vi "0_StageToStave.vi"(0 "Image feed":T1(plugin-control), 1 "Stave origin in XYZ Frame":T2, 2 "Stave Coordinate System":enum16{"Tooling Pins", "Bus Tape"}(ring), 3 "Pixel resolution [um/pix]":dbl=3.5 format="%#_13g", 4 "Axes Speeds [mm/s]":T3={"X Speed"=25.0, "Y Speed"=10.0, "Z Speed"=10.0}, 5 "N pics captured":i32=10, 6 "Pause before image capture [ms]":u32=3500, 7 "error in":errorcluster, 9 "Record keeping file path":path=path "E:/XYZstage+Camera_CollectedImages/12-22-2016/images", 11 "XYZ .NET Refnum in":refnum<k24>, 12 "Autofocus Coord in XYZ Frame":T2, 13 "Current Build Phase":refnum<vi>, 14 "Templates path":path=path "C:/Users/Sciolla Lab/Desktop/BNLStaveAssembly-Laura/edgeimagebig.png", 26 "Calibration Results":refnum<vi>) -> (15 "Cross- check: Are these the center of pins in the center of the image?":T1[](array[plugin-control])=["remote image 000000001396EDEC", "remote image 000000001392CD9C", "remote image 000000001392D204", "remote image 00000000139777D4", "remote image 000000001397783C", "image_5", "image_6", "image_7", "image_8", "image_9", "image_10", "image_11", "image_12", "image_13", "image_14", "image_15", "image_16", "image_17"], 16 "Finished!":bool, 17 "Check: Plot of average point in each pin":T4(graph), 19 "XYZ .NET Refnum out":refnum<k24>, 21 "Angle of pins [rad]":dbl, 24 "Calibrated stave origin (X,Y) [mm]":dbl[](array[numeric]), 25 "Calibrated stave basis [mm]":dbl[][](array[numeric]), 27 "Error report":errorcluster)   [LabVIEW 2016]
uses:
  C:/Users/Aerotech/Documents/BNL_ThermomechanicalStave/AerotechLibraries/Bin/Aerotech.A3200.dll
  AerotechLibraries/Bin/Aerotech.A3200.dll
  <vilib>/Utility/file.llb/Write Delimited Spreadsheet (DBL).vi
panel:
  out "Image Array":T1[](array[plugin-control])=["remote image 000000001396EDEC", "remote image 000000001392CD9C", "remote image 000000001392D204", "remote image 00000000139777D4", "remote image 000000001397783C", "image_5", "image_6", "image_7", "image_8", "image_9", "image_10", "image_11", "image_12", "image_13", "image_14", "image_15", "image_16", "image_17"]
  out "Stave Z [mm]":dbl
  out "Ideal pin locations":dbl[][](array[numeric])
  # "RESULTS"
  # "CONTROLS"
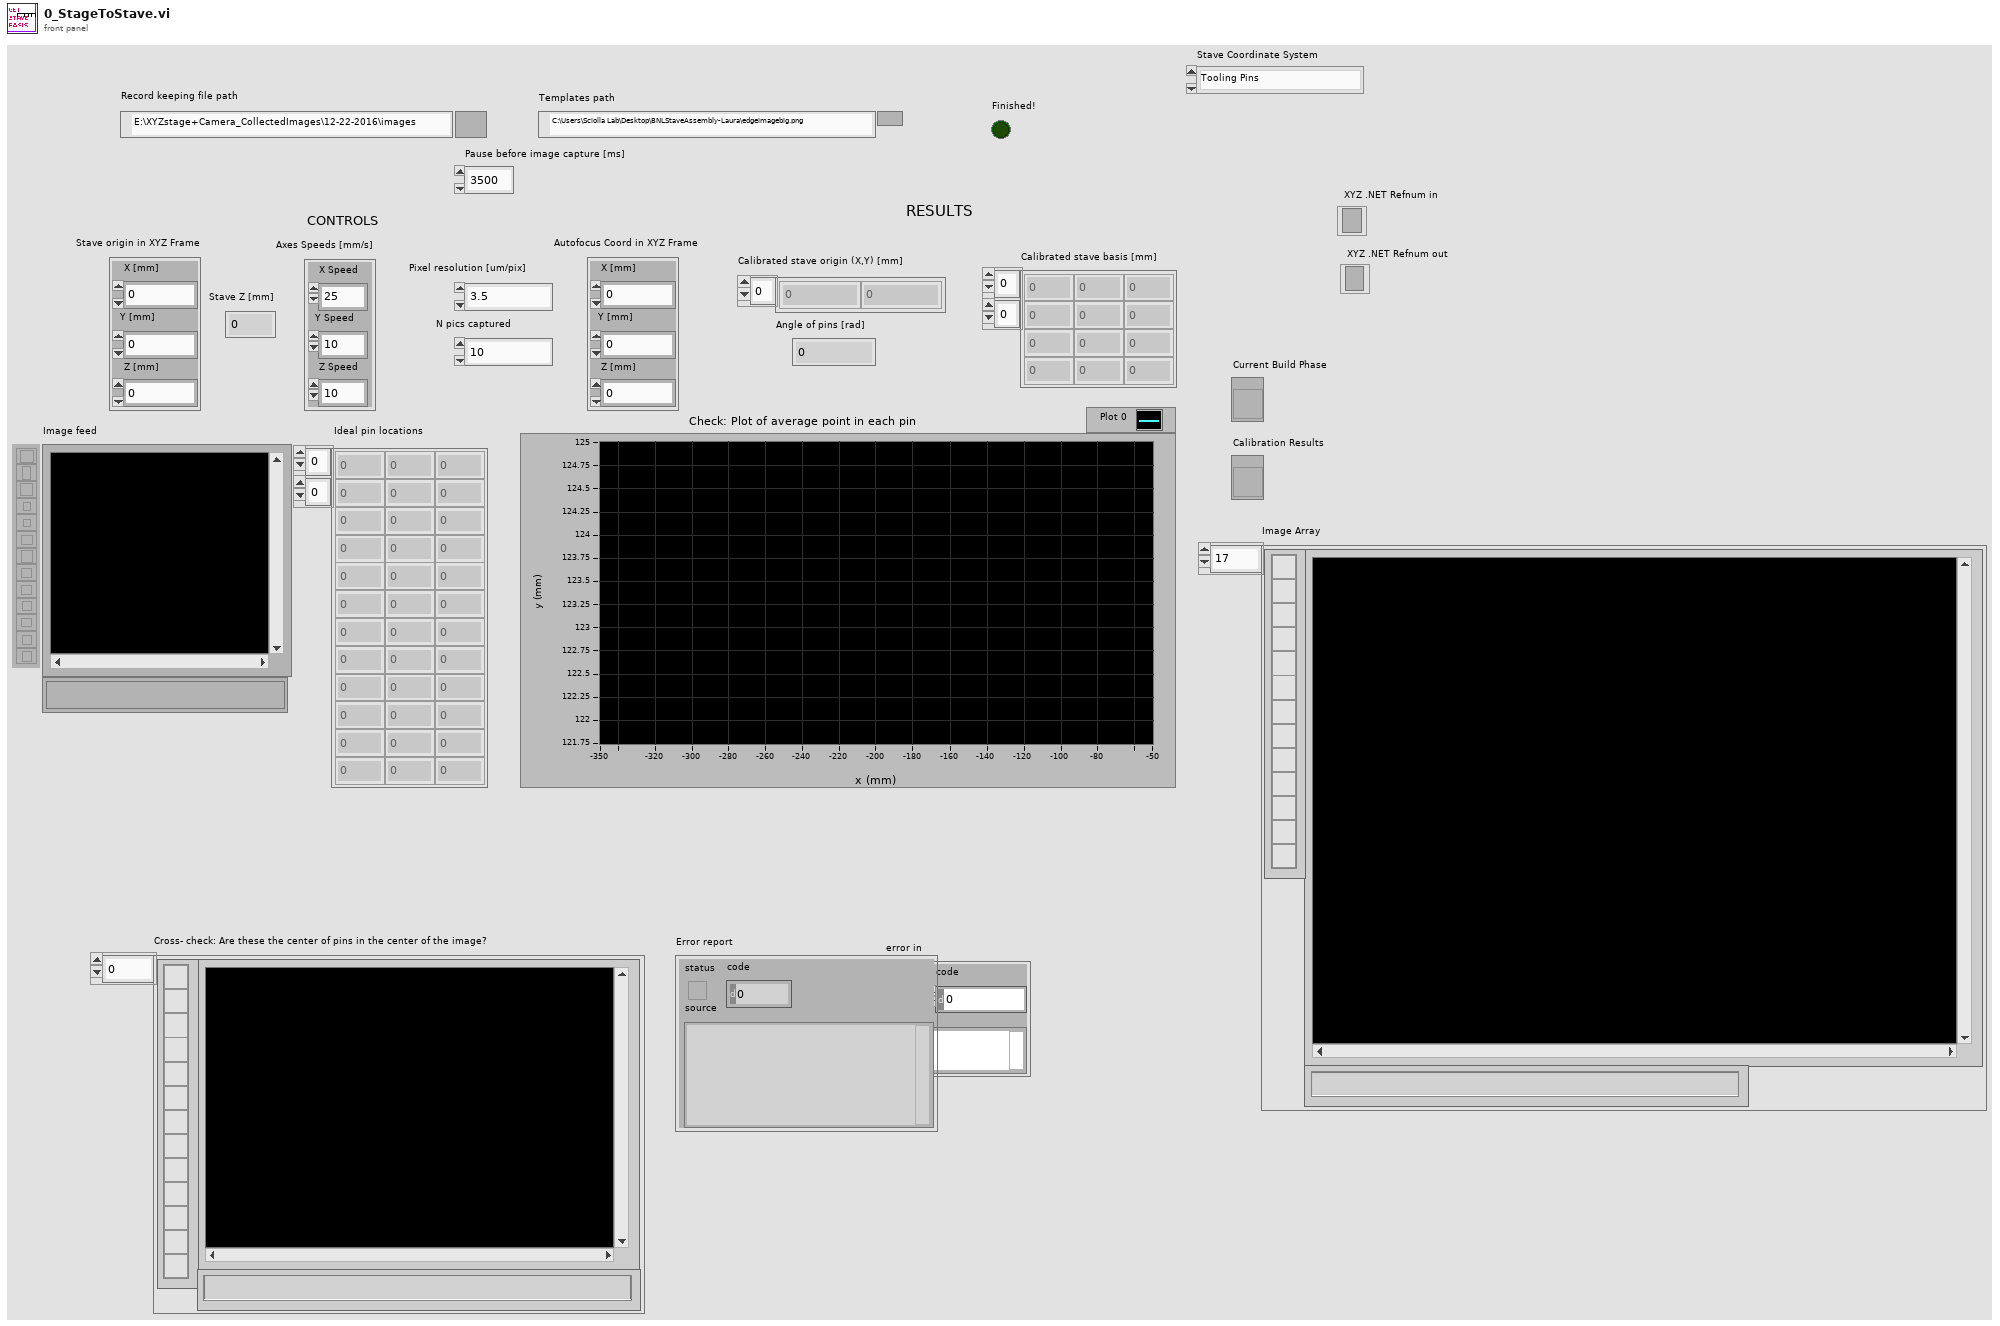
[diagram p1: front panel]
types:
  T1 = typedef "IMAQ Image.ctl" = refnum<image>
  T2 = cluster{"X [mm]":dbl, "Y [mm]":dbl, "Z [mm]":dbl}
  T3 = cluster{"X Speed":dbl, "Y Speed":dbl, "Z Speed":dbl}
  T4 = cluster{"Top averages":dbl[], "Best Linear Fit":dbl[]}[]
  T5 = cluster{"Image feed":T1, "Axes Speeds [mm/s]":cluster{"X Speed":dbl, "Y Speed":dbl, "Z Speed":dbl}, "XYZ .NET Refnum in":refnum<k24>}
  T6 = cluster{"Captured positions":dbl[][], "XYZ .NET Refnum out":refnum<k24>}
  T7 = cluster{"Camera calibration results":cluster{"Calibration [um/pix]":dbl, "Working distance to stave [mm]":dbl, "Calib uncertainty [um/pix]":dbl, "WD Uncertainty [mm]":dbl}, "Stave basis calibration results":cluster{"Angle, stave & xyz stage [rad]":dbl, "Calibrated stave origin (X,Y) [mm]":dbl[]}}
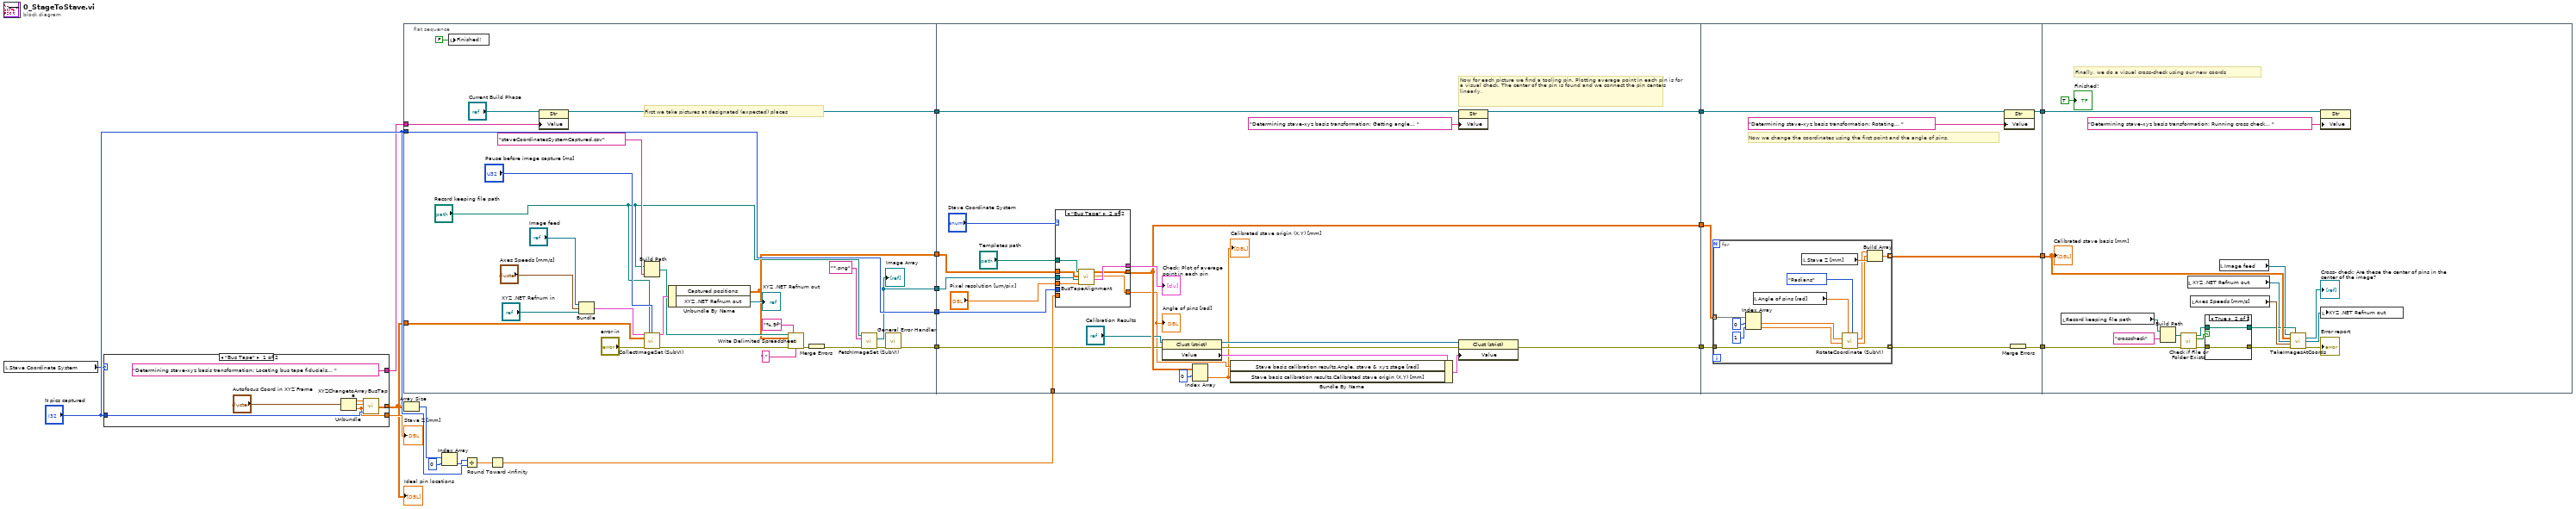
[diagram p0: block diagram]
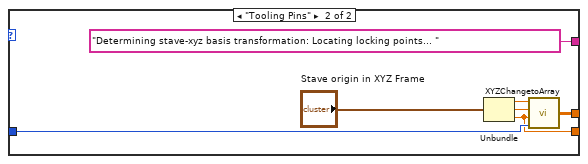
[diagram p2: hidden frame]
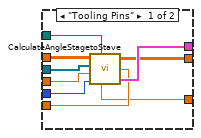
[diagram p3: hidden frame]
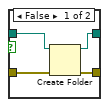
[diagram p4: hidden frame]
diagram:
  n1 = local read "Stave Coordinate System"() -> (w2:enum16{"Tooling Pins", "Bus Tape"})
  n2 = case shown="\"Bus Tape\"" w2 {
    tunnel: "N pics captured" -> [w25 w33]
    tunnel: [w23 w30] -> w8
    tunnel: [w24 w32] -> w3
    tunnel: ["Determining stave-xyz basis transformation: Locating bus tape fiducials... " ("Value") "Determining stave-xyz basis transformation: Locating locking points... " ("Value")] -> w1
    frame "Bus Tape" {
      n3 = Unbundle("Autofocus Coord in XYZ Frame") -> ("X [mm]"=w27:dbl, "Y [mm]"=w26:dbl, "Z [mm]"=w23:dbl)
      n4 = call "XYZChangetoArrayBusTape.vi"("N pics captured"=w25, "z change"=w23, "y change"=w26, "x change"=w27) -> ("Array of Coords to go to"=w24:dbl[][])  [unwired: 2 in]
    }
    frame "Tooling Pins" {
      n5 = Unbundle("Stave origin in XYZ Frame") -> ("X [mm]"=w35:dbl, "Y [mm]"=w34:dbl, "Z [mm]"=w30:dbl)
      n6 = call "XYZChangetoArray.vi"("N pics captured"=w33, "z change"=w30, "y change"=w34, "x change"=w35) -> ("Array of Coords to go to"=w32:dbl[][])  [unwired: 2 in]
    }
  }
  "Ideal pin locations" <- w3
  "Stave Z [mm]" <- w8
  n7 = flat-sequence {
    tunnel: [w43] -> w19
    tunnel: [w42] -> w17
    tunnel: [w44] -> w16
    tunnel: w3 -> [w47]
    tunnel: "N pics captured" -> [w62]
    tunnel: [w62] -> w15
    tunnel: [w59] -> w7
    tunnel: w1 -> [w37]
    tunnel: [w82] -> w21
    tunnel: w19 -> [w81]
    tunnel: [w68] -> w18
    tunnel: w17 -> [w69]
    tunnel: w16 -> [w79]
    tunnel: w15 -> [w77]
    tunnel: w9 -> [w76]
    tunnel: w7 -> [w74]
    tunnel: [w73] -> w6
    tunnel: w21 -> [w108]
    tunnel: [w107] -> w20
    tunnel: w18 -> [w103]
    tunnel: w6 -> [w105]
    tunnel: [w104] -> w5
    tunnel: [w101] -> w4
    tunnel: w20 -> [w140]
    tunnel: w5 -> [w127]
    tunnel: w4 -> [w126]
    frame #0 {
      # "First we take pictures at designated (expected) places"
      n8 = local write "Finished!"(FALSE) -> ()
      n9 = property class="Str"(reference="Current Build Phase", "Value"=w37) -> (reference out=w59:refnum<vi>)  [unwired: 1 in, 1 out]
      n10 = Bundle("Image feed"="Image feed", "Axes Speeds [mm/s]"="Axes Speeds [mm/s]", "XYZ .NET Refnum in"="XYZ .NET Refnum in") -> (w40:T5)  [unwired: 1 in]
      n11 = Build Path(base path="Record keeping file path", name or relative path="staveCoordinatesSystemCaptured.csv") -> (appended path=w50:path)
      n12 = call "CollectImageSet (SubVI).vi"("Inputs"=w40, "Path to save collected images"="Record keeping file path", "milliseconds to wait"="Pause before image capture [ms]", "Set of coordinates to process"=w47, "error in"="error in") -> ("Outputs"=w54:T6, "error out"=w56:errorcluster)  [unwired: 8 in, 1 out]
      n13 = Unbundle By Name(w54) -> ("Captured positions"=w44:dbl[][], "XYZ .NET Refnum out"=→"XYZ .NET Refnum out":refnum<k24>)
      n14 = call-poly <vilib>:"Write Delimited Spreadsheet.vi"("file path (dialog if empty)"=w50, "format (%.3f)"="%.9f", "2D data"=w44, "error in (no error)"=w56, "delimiter (\\t)"="," ("delimiter (\\t)")) -> ("error out"=w55:errorcluster)  [unwired: 9 in, 1 out]
      n15 = Merge Errors(w55) -> (w52:errorcluster)
      n16 = call "FetchImageSet (SubVI).vi"("error in (no error)"=w52, "Naming Convention"="*.png", "Images Directory"="Record keeping file path") -> ("error out"=w51:errorcluster, "Image Array"=w43:T1[])  [unwired: 6 in, 1 out]
      "Image Array" <- w43
      n17 = call <vilib>:"General Error Handler.vi"("error in (no error)"=w51) -> ("error out"=w42:errorcluster)  [unwired: 2 in, 12 out]
    }
    frame #1 {
      # "Now for each picture we find a tooling pin. Plotting average point in each pin is for a visual check. The center of the pin is found and we connect the pin centers linearly."
      n18 = case shown="\"Bus Tape\"" "Stave Coordinate System" {
        tunnel: [w93 w96] -> w84
        tunnel: [w92 w95] -> w82
        tunnel: w81 -> [w91 w98]
        tunnel: "Pixel resolution [um/pix]" -> [w90 w97]
        tunnel: w79 -> [w89 w99]
        tunnel: "Templates path" -> [w88 w100]
        tunnel: w77 -> [w87 _]
        tunnel: w76 -> [w86 _]
        tunnel: [w85 w94] -> w66
        frame "Tooling Pins" {
          n19 = call "CalculateAngleStagetoStave.vi"("Coordinates from images"=w89, "Templates path"=w88, "Image Array"=w91, "Pixel resolution"=w90, "Number of images each"=w87, "Number of pins"=w86) -> ("Angle"=w85:dbl, "Locations pins"=w92:dbl[][], "Each point on located edges"=w93:T4)
        }
        frame "Bus Tape" {
          n20 = call "BusTapeAlignment.vi"("um/pix resolution"=w97, "Input Images Array"=w98, "Input Coordinate Array"=w99, "Template Path"=w100) -> ("Bus Tape Positions"=w96:cluster{"Top":dbl[], "Top":dbl[]}[], "Angle (rad)"=w94:dbl, "Average positions"=w95:dbl[][])  [unwired: 4 in, 1 out]
        }
      }
      "Check: Plot of average point in each pin" <- w84
      "Angle of pins [rad]" <- w66
      n21 = property class="Clust (strict)"(reference="Calibration Results", error in=w69) -> (reference out=w71:refnum<vi>, error out=w70:errorcluster, "Value"=w67:T7)
      n22 = Index Array(array=w82, index (row)=0) -> (element=w65:dbl[])  [unwired: 1 in]
      "Calibrated stave origin (X,Y) [mm]" <- w65
      n23 = Bundle By Name(cluster=w67, "Stave basis calibration results.Angle, stave & xyz stage [rad]"=w66, "Stave basis calibration results.Calibrated stave origin (X,Y) [mm]"=w65) -> (w64:T7)
      n24 = property class="Str"(reference=w74, "Value"="Determining stave-xyz basis transformation: Getting angle... ") -> (reference out=w73:refnum<vi>)  [unwired: 1 in, 1 out]
      n25 = property class="Clust (strict)"(reference=w71, error in=w70, "Value"=w64) -> (error out=w68:errorcluster)  [unwired: 1 out]
    }
    frame #2 {
      # "Now we change the coordinates using the first point and the angle of pins."
      n26 = for {
        tunnel: w108 -> [w119] mode=indexing
        tunnel: [w116] -> w107 mode=indexing
        tunnel: w103 -> [w110]
        tunnel: [w109] -> w102 mode=indexing
        n27 = Index Array(array=w119, index #1=0 ("index"), index #2=1 ("index")) -> (element #1=w112:dbl, element #2=w111:dbl)
        n28 = local read "Angle of pins [rad]"() -> (w121:dbl)
        n29 = local read "Stave Z [mm]"() -> (w115:dbl)
        n30 = call "RotateCoordinate (SubVI).vi"("Units"=enum16{"mrad", "Radians", "Degrees"}."Radians", "Angle"=w121, "error in (no error)"=w110, "y"=w111, "x"=w112) -> ("error out"=w109:errorcluster, "y'"=w114:dbl, "x'"=w113:dbl)  [unwired: 4 in]
        n31 = Build Array(w113, w114, w115) -> (w116:dbl[])
      }
      n32 = property class="Str"(reference=w105, "Value"="Determining stave-xyz basis transformation: Rotating... ") -> (reference out=w104:refnum<vi>)  [unwired: 1 in, 1 out]
      n33 = Merge Errors(w102) -> (w101:errorcluster)
    }
    frame #3 {
      # "Finally, we do a visual cross-check using our new coords"
      n34 = local read "Record keeping file path"() -> (w136:path)
      n35 = Build Path(base path=w136, name or relative path="crosscheck") -> (appended path=w134:path)
      n36 = call <vilib>:"Check if File or Folder Exists.vi"("error in (no error)"=w126, "path"=w134) -> ("error out"=w131:errorcluster, "file or folder exists?"=w133:bool, "dup path"=w132:path)  [unwired: 7 in]
      n37 = local read "XYZ .NET Refnum out"() -> (w123:refnum<k24>)
      n38 = local read "Axes Speeds [mm/s]"() -> (w139:T3)
      n39 = case shown="True" w133 {
        tunnel: w132 -> [w144 w146]
        tunnel: [w143 w146] -> w125
        tunnel: w131 -> [w142 w145]
        tunnel: [w141 w145] -> w130
        frame False {
          n40 = Create Folder(path (use dialog)=w144, error in=w142) -> (created path=w143:path, error out=w141:errorcluster)  [unwired: 1 in, 1 out]
        }
        frame True {
        }
      }
      n41 = local read "Image feed"() -> (w122:T1)
      n42 = call "TakeImagesAtCoords.vi"("Image feed"=w122, "Path to save stave calib"=w125, "Set of Coordinates to Process"=w140, "XYZ .NET Refnum in"=w123, "Axes Speeds [mm/s]"=w139, "error in"=w130) -> ("Image Array"=→"Cross- check: Are these the center of pins in the center of the image?":T1[], "XYZ .NET Refnum out"=w124:refnum<k24>, "Error report"=→"Error report":errorcluster)  [unwired: 6 in, 1 out]
      n43 = property class="Str"(reference=w127, "Value"="Determining stave-xyz basis transformation: Running cross check... ") -> ()  [unwired: 1 in, 2 out]
      n44 = local write "XYZ .NET Refnum out"(w124) -> ()
      "Calibrated stave basis [mm]" <- w140
      "Finished!" <- TRUE ("Finished!")
    }
  }
  n45 = Array Size(array=w3) -> (size(s)=w14:i32[])
  n46 = Index Array(array=w14, index=0) -> (element=w11:i32)
  n47 = Divide(x=w11, y="N pics captured") -> (x/y=w10:dbl)
  n48 = Round Toward -Infinity(1:w10) -> (0:w9:dbl)
